vi "Create Log File.vi"(4 "rollover":enum32{"hourly", "daily"}(radio), 6 "create new":bool, 8 "error in (no error)":errorcluster, 9 "name prefix":string, 10 "Directory":path, 11 "file reference in":refnum<file>) -> (0 "error out":errorcluster, 3 "file reference out":refnum<file>)   [LabVIEW 2024]
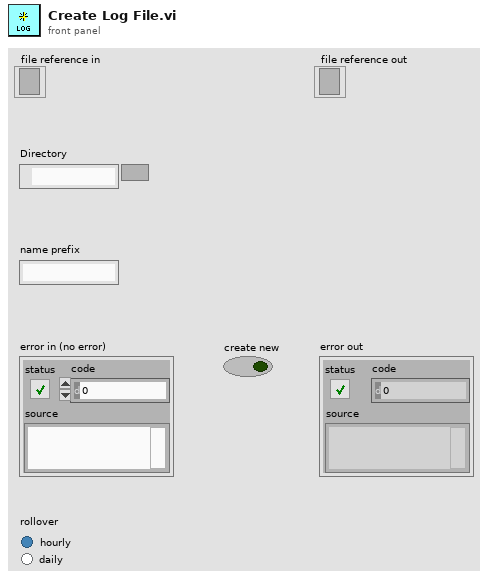
[diagram p1: front panel]
types:
  T1 = typedef "LVDateTimeRec.ctl" = cluster{"fractional second":dbl, "second":i32, "minute":i32, "hour":i32, "day of month":i32, "month":i32, "year":i32, "day of week":i32, "day of year":i32, "DST":i32}
  T2 = enum16{"open", "replace", "create", "open or create", "replace or create", "replace or create with confirmation"}
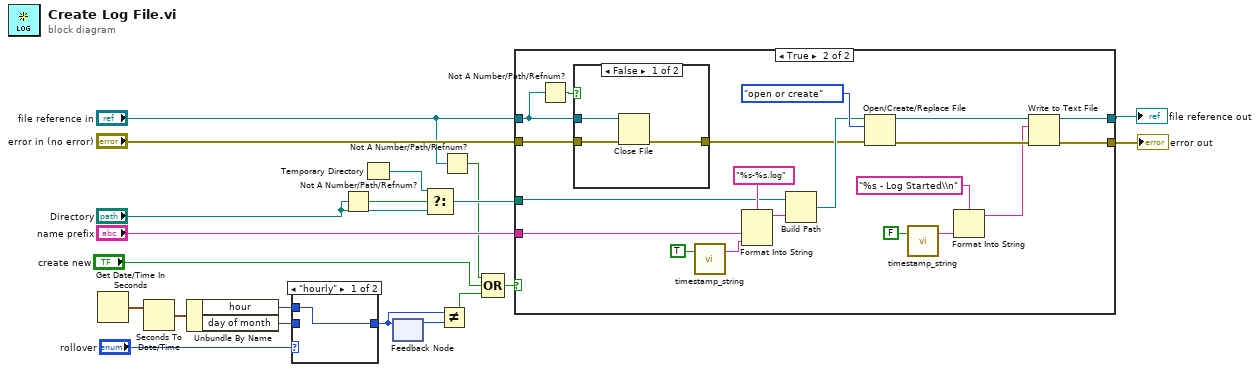
[diagram p0: block diagram]
diagram:
  n1 = Get Date/Time In Seconds() -> (seconds since 1Jan1904=w9:timestamp)
  n2 = Seconds To Date/Time(time stamp (now)=w9) -> (date time rec=w8:T1)  [unwired: 1 in]
  n3 = Unbundle By Name(w8) -> ("hour"=w5:i32, "day of month"=w6:i32)
  n4 = case shown="\"hourly\"" "rollover" {
    tunnel: [w21 w22] -> w3
    tunnel: w6 -> [_ w22]
    tunnel: w5 -> [w21 _]
    frame "hourly" {
    }
    frame "daily" {
    }
  }
  n5 = Not A Number/Path/Refnum?(number/path/refnum="Directory") -> (NaN/Path/Refnum?=w20:bool)
  n6 = Temporary Directory() -> (w19:path)
  n7 = feedback-in #1(w3) -> ()
  n8 = feedback #1() -> (w4:i32)  [unwired: 1 in]
  n9 = Select(t=w19, s=w20, f="Directory") -> (s? t:f=w17:path)
  n10 = Not Equal?(x=w3, y=w4) -> (x != y?=w2:bool)
  n11 = Not A Number/Path/Refnum?(number/path/refnum="file reference in") -> (NaN/Path/Refnum?=w10:bool)
  n12 = Compound Arithmetic op=OR(w10, "create new", w2) -> (w11:bool)
  n13 = case shown="True" w11 {
    tunnel: w17 -> [_ w41]
    tunnel: "name prefix" -> [_ w42]
    tunnel: [w24 w31] -> w15
    tunnel: "file reference in" -> [w24 w37]
    tunnel: "error in (no error)" -> [w23 w35]
    tunnel: [w23 w29] -> w13
    frame False {
    }
    frame True {
      n14 = Not A Number/Path/Refnum?(number/path/refnum=w37) -> (NaN/Path/Refnum?=w38:bool)
      n15 = case shown="False" w38 {
        tunnel: w37 -> [w47 _]
        tunnel: [w46 w48] -> w36
        tunnel: w35 -> [w45 w48]
        frame False {
          n16 = Close File(refnum=w47, error in=w45) -> (error out=w46:errorcluster)  [unwired: 1 out]
        }
        frame True {
        }
      }
      n17 = call "timestamp_string.vi"("make file friendly"=TRUE) -> ("timestamp string"=w34:string)  [unwired: 2 in]
      n18 = Format Into String(format string="%s-%s.log" ("Following RFC 3339 (ISO8601)"), w42, w34) -> (resulting string=w40:string)  [unwired: 2 in, 1 out]
      n19 = Build Path(base path=w41, name or relative path=w40) -> (appended path=w39:path)
      n20 = Open/Create/Replace File(file path (use dialog)=w39, error in=w36, operation (0:open)=T2."open or create") -> (refnum out=w32:refnum<file>, error out=w30:errorcluster)  [unwired: 3 in, 1 out]
      n21 = call "timestamp_string.vi"("make file friendly"=FALSE) -> ("timestamp string"=w26:string)  [unwired: 2 in]
      n22 = Format Into String(format string="%s - Log Started\\n", w26) -> (resulting string=w25:string)  [unwired: 2 in, 1 out]
      n23 = Write to Text File(file (use dialog)=w32, text=w25, error in=w30) -> (refnum out=w31:refnum<file>, error out=w29:errorcluster)  [unwired: 1 in, 1 out]
    }
  }
  "file reference out" <- w15
  "error out" <- w13
